vi "2DScatterFit2.vi"() -> ()   [LabVIEW 2014]
uses:
  <vilib>/Analysis/1siggen.llb/Ramp Pattern by Samples.vi
  <vilib>/gmath/NumericalOptimization/Nonlinear Curve Fit LM.vi
  <vilib>/Platform/NI_3dgraph.lvlib
  <vilib>/gmath/NI_Gmath.lvlib
  <vilib>/Analysis/NI_AALBase.lvlib
panel:
  in  "View":enum32{"2D", "3D"}(tab)=enum."3D"
  out "Z, Fit/Guess, Residual":dbl[][](graph)
  out "X,Y":dbl[][](graph)
  in  "3D Curve":refnum<k7>(container)
  in  "Fit!":bool
  out "Best Fit":dbl[](array[numeric]) format="%.2f"
  in  "Guess":dbl[](array[numeric])=[3.0, 10.0, -2.0, 10.0, 5.0] format="%.2f"
  out "Parameter Names":string[](array[string])=["Xposition", "Xwidth", "Yposition", "Ywidth", "Amplitude"]
  in  "stop":bool
  out "note":string
  # "Demo for NI-WEEK 2007\nChristian Altenbach\naltenbach@gmail.com"
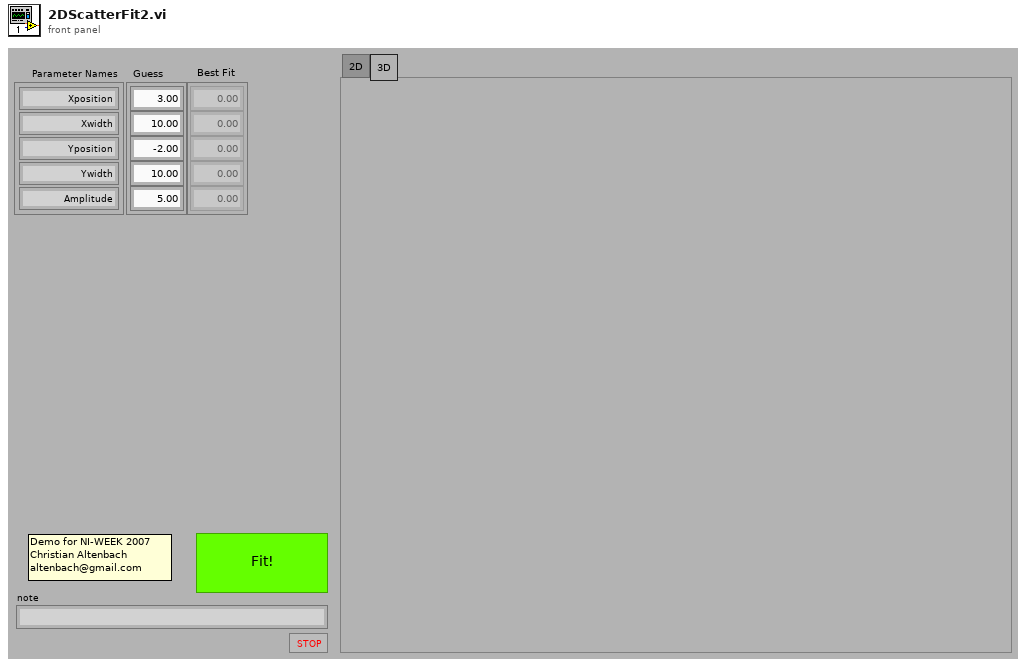
[diagram p1: front panel]
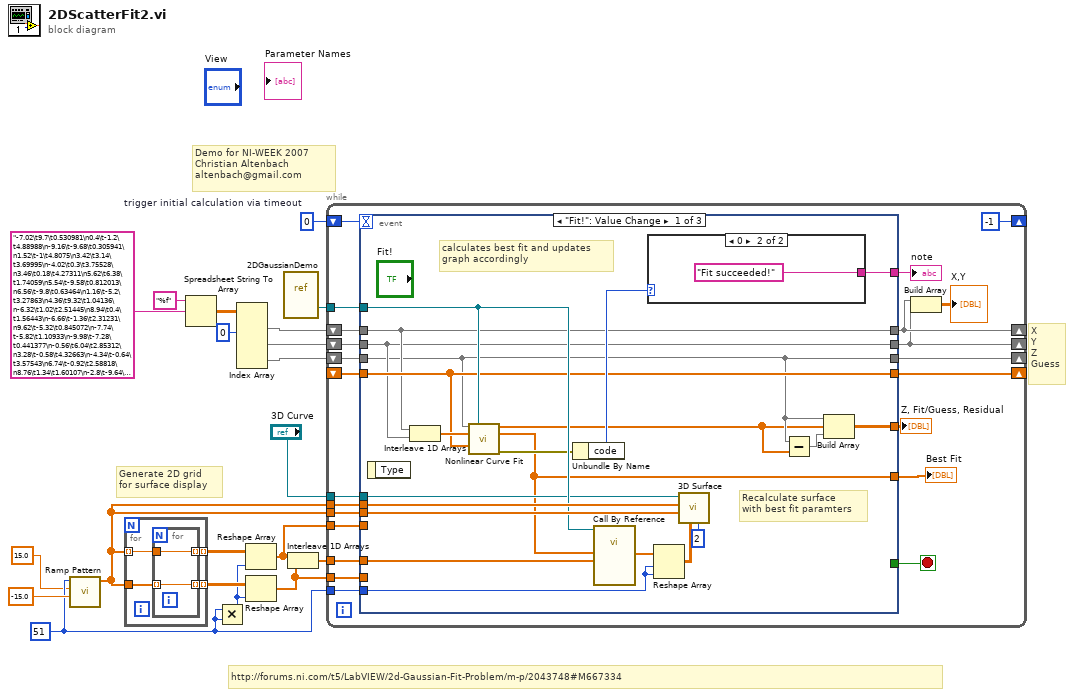
[diagram p0: block diagram]
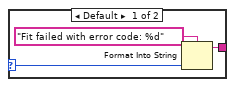
[diagram p2: hidden frame]
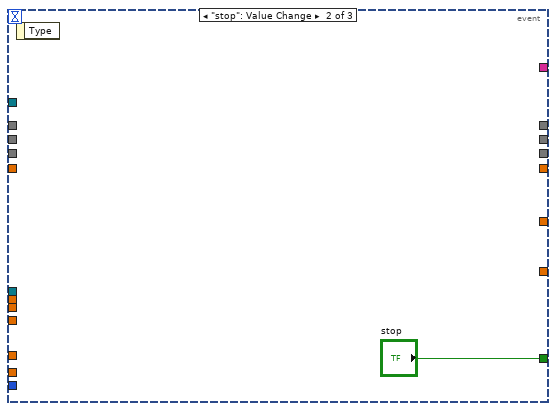
[diagram p3: hidden frame]
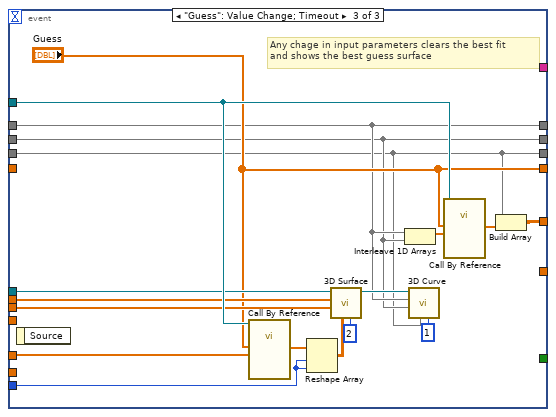
[diagram p4: hidden frame]
diagram:
  w14 = 0  # trigger initial calculation via timeout
  w16 = 51 ("samples")
  # "http://forums.ni.com/t5/LabVIEW/2d-Gaussian-Fit-Problem/m-p/2043748#M667334"
  # "Demo for NI-WEEK 2007\nChristian Altenbach\naltenbach@gmail.com"
  # "X\nY\nZ\nGuess"
  # "Generate 2D grid\nfor surface display"
  n1 = call-poly <vilib>:"Ramp Pattern.vi"("start"=-15.0, "end"=15.0, "samples"=w16) -> ("Ramp Pattern"=w8:dbl[])  [unwired: 7 in, 1 out]
  n2 = for {
    tunnel: w8 -> [w24] mode=indexing
    tunnel: w8 -> [w23]
    tunnel: [w22] -> w19 mode=indexing
    tunnel: [w21] -> w18 mode=indexing
    n3 = for {
      tunnel: w24 -> [w26]
      tunnel: w23 -> [w25] mode=indexing
      tunnel: [w26] -> w22 mode=indexing
      tunnel: [w25] -> w21 mode=indexing
    }
  }
  n4 = Spreadsheet String To Array(format string="%f", spreadsheet string="-7.02\t9.7\t0.530981\n0.4\t-1.2\t4.88988\n-9.16\t-9.68\t0.305941\n1.52\t-1\t4.8075\n3.42\t3.14\t3.69995\n-4.02\t0.3\t3.75528\n3.46\t0.18\t4.27311\n5.62\t6.38\t1.74059\n5.54\t-9.58\t0.812013\n6.56\t-9.8\t0.63464\n1.16\t-5.2\t3.27863\n4.36\t9.32\t1.04136\n-6.32\t1.02\t2.51445\n8.94\t0.4\t1.56443\n-6.66\t-1.36\t2.31231\n9.62\t-5.32\t0.845072\n-7.74\t-5.82\t1.10933\n-9.98\t-7.28\t0.441377\n-0.56\t6.04\t2.85312\n3.28\t-0.58\t4.32663\n-4.34\t-0.64\t3.57543\n6.74\t-0.92\t2.58818\n8.76\t1.34\t1.60107\n-2.8\t-9.64\t1.05793\n8.26\t-4.1\t1.44729\n5.88\t1.34\t2.99639\n0.68\t-1.06\t4.90224\n-6.74\t4.42\t1.7417\n4.4\t-6.82\t1.90029\n4.36\t-8.66\t1.24117\n4.62\t3.24\t3.18956\n3.4\t8.42\t1.47493\n8.46\t-9.42\t0.46356\n9.06\t-8.98\t0.447721\n-0.1\t8.6\t1.63387\n9.4\t-0.78\t1.36902\n-5.2\t-2.52\t2.85715\n-3.18\t-7.78\t1.66237\n-4.08\t-0.64\t3.70658\n3.18\t3.78\t3.53928\n7.86\t-6.78\t1.02478\n-5.44\t-3.16\t2.59411\n-7.94\t9.98\t0.391925\n6.6\t-1.12\t2.64428\n1.96\t7.26\t2.16044\n-0.86\t-3.3\t4.15442\n-2.28\t4.72\t3.23096\n-8.48\t-8.54\t0.507106\n1.48\t-1.14\t4.79288\n-2.56\t-6.28\t2.42944\n-7.78\t-1.96\t1.73096\n-0.12\t-1.6\t4.79692\n0.82\t-2.54\t4.51213\n6.32\t-0.22\t2.84146\n4.98\t-5.72\t2.16342\n3.52\t6.54\t2.22911\n4.34\t2.46\t3.53708\n-7.36\t-3.3\t1.72222\n-4.66\t7.86\t1.35106\n4.28\t-7.26\t1.75649\n6.4\t3.18\t2.40575\n-6.7\t-3.58\t1.94133\n-7.3\t3.08\t1.78659\n-5.94\t3.94\t2.1791\n-8.62\t-1\t1.45051\n-4.82\t0.8\t3.31652\n-3.58\t-5.66\t2.44563\n-5.26\t-3.06\t2.70188\n-6.32\t-0.66\t2.53662\n-4.84\t1.68\t3.19938\n-4.1\t6.08\t2.13012\n-1.78\t-1.34\t4.55738\n-2.32\t3.54\t3.73108\n0.1\t0.96\t4.92949\n-9.52\t-7.42\t0.493349\n6.34\t5.98\t1.65203\n-2.3\t0.98\t4.44901\n6.88\t-9.5\t0.649987\n9.6\t-1.72\t1.24779\n-9.04\t5.76\t0.793552\n-1.82\t-8.98\t1.37785\n2.34\t-7.8\t1.86285\n-7.5\t-2.46\t1.79252\n-6\t-5.16\t1.81762\n-6.56\t3.08\t2.10648\n3.4\t-2.04\t4.03612\n8.72\t-5.28\t1.08912\n7.32\t0.18\t2.32211\n7.92\t-3.52\t1.67987\n-3.08\t9.6\t1.04529\n-2.5\t4.24\t3.38577\n-7.24\t-1.42\t2.02639\n-4.1\t0.66\t3.69618\n-0.22\t-1.02\t4.90226\n8.32\t-9.62\t0.453237\n2.26\t-3.06\t4.08115\n1.84\t-5.08\t3.2556\n-1.16\t8.06\t1.81703\n0.48\t7.64\t2.07089\n-2.38\t-7.86\t1.75913\n0.08\t8.72\t1.58589\n-9.02\t8.62\t0.428851\n3.4\t0.26\t4.29596\n-9.24\t-8.94\t0.368135\n-5\t1.34\t3.16682\n3.14\t2.58\t3.9853\n-3.6\t2.74\t3.5415\n3.58\t-9.46\t1.08953\n0.98\t2.2\t4.61388\n-7.94\t1.82\t1.67746\n8.94\t-0.64\t1.55819\n7.92\t-2.48\t1.84647\n2.38\t-9.32\t1.25331\n4.74\t8.24\t1.31895\n0.32\t4.56\t3.65473\n5.64\t8.84\t0.9855\n-6.42\t-3.82\t2.0049\n-2.02\t-6.38\t2.48753\n-0.06\t2.68\t4.4803\n8.64\t-8.68\t0.542172\n-1.02\t-1.96\t4.59522\n-1.3\t-0.04\t4.81179\n7.2\t8.12\t0.881388\n-1.24\t1.92\t4.56605\n-7.1\t5.64\t1.33583\n3.76\t-0.96\t4.08675\n-8.6\t5.22\t0.982076\n7.96\t7.5\t0.859444\n-0.2\t-1.66\t4.77755\n0\t-7.24\t2.25744\n-8\t8.4\t0.598539\n-2\t4.88\t3.22355\n-6.04\t5.56\t1.69424\n4.36\t-6.98\t1.84718\n-1.64\t1.98\t4.45456\n0.84\t0.98\t4.90476\n-0.18\t6.64\t2.5628\n3.66\t1.7\t4.01154\n9.84\t0.36\t1.21478\n-1.68\t-7.36\t2.07473\n-8.28\t-9.08\t0.463232\n-5.22\t-9.38\t0.8276\n-4.22\t7.96\t1.40648\n2.34\t6.82\t2.32071\n-5.94\t-2.14\t2.56781\n4.66\t1.72\t3.55425\n-4.4\t-0.94\t3.51923\n-5.26\t0.28\t3.11132\n1.22\t-3.22\t4.21313\n-9.94\t6.84\t0.492513\n-1.34\t-1.88\t4.55075\n7.44\t-0.02\t2.26275\n-2.46\t7.1\t2.08189\n-2.02\t7.84\t1.823\n4.36\t-0.5\t3.84916\n2.26\t2.78\t4.18858\n-2.58\t-1.9\t4.1725\n5.22\t-3.4\t2.87572\n2.02\t7.56\t2.01372\n-8.9\t-4.5\t1.00198\n5.26\t9.28\t0.928388\n-1.34\t-4.98\t3.29733\n-8.96\t-3.36\t1.12821\n-4.14\t-4.92\t2.56328\n-4.66\t9.92\t0.776929\n-4.82\t-5.04\t2.278\n0.84\t-8.86\t1.5156\n8.42\t8.38\t0.621874\n-7.86\t-0.58\t1.78954\n1.68\t-1.68\t4.64565\n-9.28\t5.52\t0.77081\n-9.44\t-7.76\t0.467417\n1.78932e-307\t7.18\t2.29428\n-5\t-3.06\t2.82177\n-9.88\t4.02\t0.796954\n-5.74\t-6.44\t1.52521\n-6.74\t-7.48\t1.00177\n2.04\t-7.3\t2.12571\n-1.6\t1.08\t4.65393\n1.38\t9.28\t1.33725\n-3.64\t4.9\t2.74756\n-0.34\t-2.5\t4.52021\n4.9\t1.08\t3.53143\n3.74\t6.14\t2.35232\n3.64\t3.62\t3.44611\n-5.26\t-6.82\t1.53957\n9.04\t-1.62\t1.46654\n3.26\t1.1\t4.27932\n9.46\t-1.92\t1.28447\n4.18\t-8.36\t1.37098\n0.12\t-2.64\t4.49572\n-8.22\t1.04\t1.61376\n-1.82\t7.7\t1.90962\n-5.2\t-5.24\t2.07535\n-2.4\t-7.62\t1.8578\n-8.78\t2.8\t1.25228\n4.24\t1.76\t3.74421\n3.54\t-5.6\t2.63663\n-9.2\t7.88\t0.489488\n-6.56\t-6.74\t1.22082\n-8.04\t-0.3\t1.71602\n-2.8\t-7.58\t1.80952\n-0.84\t-1.86\t4.65302\n0.32\t9.36\t1.33229\n-4.24\t-9.12\t1.0357\n-7.3\t0.76\t2.04315\n-8.02\t7.6\t0.7225\n3.72\t-2.14\t3.88248\n-0.02\t-5.3\t3.26176\n-3.06\t1.22\t4.118\n8.7\t-9.42\t0.43588\n5.5\t-4.28\t2.48422\n-1\t0.5\t4.85807\n6.78\t5.7\t1.59355\n-1.38\t-8.48\t1.61302\n-2.46\t9.8\t1.04498\n-2.8\t7.68\t1.77408\n9.06\t-3.94\t1.19958\n1.18\t4.78\t3.49872\n1.76\t-3.06\t4.19197\n8.98\t5.58\t0.970049\n0.64\t4.22\t3.81545\n5.74\t-5.32\t2.05272\n10\t4.06\t0.905243\n-1.36\t-6.42\t2.56925\n8.48\t-8\t0.670589\n-8.36\t-4.34\t1.18762\n4.12\t8.04\t1.50018\n0.62\t1.12\t4.89826\n9.38\t-8.68\t0.44404\n8.32\t-7.94\t0.708242\n-4\t-4.34\t2.83319\n-0.7\t7.52\t2.09889\n-9.78\t4.08\t0.816216\n-4.92\t-1.72\t3.15008\n7.58\t3.94\t1.73579\n9.04\t2.14\t1.42498\n7.96\t2.06\t1.88441\n1.36\t-1.34\t4.77709\n-9.38\t-0.36\t1.18229\n-5.84\t4.38\t2.10161\n9.36\t7.22\t0.63646\n6.5\t7.62\t1.14429\n7.12\t-0.32\t2.42109\n9.16\t3.62\t1.21274\n-8.66\t-8.64\t0.470379\n-0.14\t9.5\t1.27683\n8.88\t-9.08\t0.457232\n-1.74\t-0.8\t4.64992\n0.82\t-3.56\t4.10614\n0.86\t-1.34\t4.83907\n-2.26\t-9.74\t1.07659\n-4.04\t0.56\t3.73287\n-5.4\t-5.74\t1.84518\n-1.16\t-0.48\t4.82604\n5.68\t4.6\t2.31489\n6.6\t7.04\t1.27612\n-0.38\t6.78\t2.48257\n-6.82\t6.44\t1.229\n-5.52\t-9.28\t0.807905\n4.52\t7.98\t1.44792\n-7.3\t5.78\t1.24511\n-6.72\t3.78\t1.89343\n-3.94\t-4.42\t2.82543\n-5.88\t2.8\t2.47513\n0.76\t-6.82\t2.46242\n-1.5\t5.92\t2.80718\n-7.7\t-4\t1.46848\n9.8\t0.86\t1.21804\n0.66\t0.88\t4.93146\n-1.8\t-2.76\t4.16679\n-4.94\t-1.08\t3.22664\n-4.14\t1.54\t3.5708\n-0.74\t-9.32\t1.32085\n-8.24\t-7.9\t0.633937\n6.24\t1.16\t2.82878\n6.78\t-5.8\t1.56221\n-6.58\t-5.46\t1.53981\n8.6\t-5.08\t1.15931\n-2.34\t9.62\t1.11263\n6.86\t-1.76\t2.44135\n-9.94\t-5.7\t0.609686\n8.04\t0.04\t1.97037\n-8.76\t1.12\t1.39063\n-9.54\t3.04\t0.982464\n6.08\t1.84\t2.82423\n-0.56\t-8.18\t1.79549\n-1.14\t2.62\t4.37226\n2.04\t7.94\t1.84031\n8.28\t-1\t1.83024\n2.24\t4.7\t3.3766\n2.36\t-9.08\t1.34164\n-4.1\t2.34\t3.42625\n-6.46\t-2.3\t2.28934\n5.78\t2.98\t2.7396\n-6.38\t-7.04\t1.19061\n-3.56\t5.6\t2.48263\n8.8\t-0.2\t1.62641\n9.44\t1.06\t1.34367\n-5.46\t5.62\t1.86836\n-1.96\t7.1\t2.16336\n-9.16\t-2.82\t1.12022\n2.56\t3.32\t3.90749\n-3\t-4.32\t3.19202\n5.08\t6.22\t1.95291\n6.66\t-8.32\t0.933789\n4.58\t4.14\t2.90085\n2.86\t0.12\t4.50896\n-8.1\t-7.7\t0.689307\n-6.98\t-4.78\t1.56816\n4.84\t7.9\t1.41309\n3.98\t5.76\t2.4525\n2.92\t4.8\t3.17122\n-3.14\t9.7\t1.0089\n2.7\t8.94\t1.36649\n2.24\t9.48\t1.21308\n-7.52\t-7\t0.931012\n-4.98\t6.9\t1.59128\n7.56\t-8.36\t0.764436\n9.56\t-1.86\t1.25265\n5\t-3.66\t2.89028\n-5.6\t8.78\t0.916387\n-1.22\t-9.58\t1.20359\n7.74\t8.68\t0.678151\n-5.22\t4.18\t2.41026\n-8.14\t7.16\t0.772657\n5.76\t9.68\t0.763586\n8.7\t7.9\t0.651396\n6.28\t-4.12\t2.2145\n-5.7\t3.94\t2.27983\n7.86\t3.7\t1.6732\n-5.7\t-7.32\t1.27926\n-6.2\t0.82\t2.59037\n-1.42\t-9.04\t1.38761\n-5.6\t-3.12\t2.53047\n-3.56\t9.98\t0.885656\n1.78\t-1.62\t4.63875\n-8.46\t-9.82\t0.357291\n4.88\t3.64\t2.95183\n-3.04\t-3.42\t3.5328\n4.56\t-2.08\t3.52554\n-9.9\t-6.6\t0.522166\n8.56\t8.34\t0.606263\n7.8\t-0.6\t2.07371\n6.5\t-1.16\t2.69229\n1.14\t2.56\t4.47883\n4.86\t5.32\t2.35856\n-9.28\t-4.7\t0.873001\n2\t-9.52\t1.21076\n1.5\t9.48\t1.25812\n3.16\t-1.02\t4.3274\n-2.28\t-8.84\t1.38434\n-4.58\t-7.74\t1.40204\n-1.94\t-4\t3.63595\n2.82\t3.72\t3.67302\n-9.42\t3.88\t0.933114\n1.18\t-6.48\t2.61318\n7.74\t-5.94\t1.23873\n-6.78\t3.88\t1.84746\n1.26\t0.28\t4.92015\n3.6\t-6.34\t2.29253\n-2.66\t5.56\t2.7461\n-6.26\t-6.2\t1.44374\n-8.46\t-2.72\t1.3749\n-2.94\t2.06\t3.99896\n3.8\t2.3\t3.81171\n-6.24\t-2.04\t2.43612\n-6.64\t1.76\t2.28036\n5.98\t-1.96\t2.85279\n-6.06\t6.2\t1.50633\n-7.36\t-9.36\t0.53925\n8.62\t-9.48\t0.437436\n4.7\t-9\t1.08385\n4.72\t9.12\t1.05003\n-0.22\t-3.74\t4.0284\n9.12\t-9.46\t0.385258\n-2.44\t0.38\t4.45242\n2.92\t-7.1\t2.09124\n-5.48\t9.22\t0.830769\n-3.28\t-1.36\t3.99856\n-1\t-4.54\t3.56697\n5.48\t9.54\t0.832893\n6.28\t-6.2\t1.60008\n3.42\t1.7\t4.10981\n-6.62\t-4.32\t1.80755\n-0.78\t0.76\t4.87278\n-5.64\t4.48\t2.15221\n-9.04\t-3.42\t1.09587\n-4.94\t-9.62\t0.809049\n1.06\t-1.5\t4.78549\n8.22\t5.58\t1.17943\n-8.7\t-9.84\t0.332602\n8.44\t-1.04\t1.75636\n-2.14\t4.68\t3.28446\n7.18\t-8.56\t0.789354\n6.3\t-0.62\t2.83738\n7.84\t-9.24\t0.567122\n6.52\t-8.92\t0.820607\n0.62\t6.54\t2.6179\n7.82\t-9\t0.608791\n-2.34\t5.22\t2.98308\n-6.16\t-0.32\t2.63306\n7.96\t5.18\t1.34015\n-2.28\t2.02\t4.25171\n-7.7\t-8.38\t0.64629\n-3.2\t2.3\t3.83204\n-1.5\t-8.3\t1.67774\n7.92\t-0.8\t2.00762\n-3.86\t9.44\t1.00007\n2.2\t0.8\t4.67731\n-8.32\t0.6\t1.58881\n0.24\t-0.52\t4.97894\n3.54\t7.98\t1.62222\n6.94\t7.08\t1.18185\n-3.14\t-3.88\t3.32287\n6.6\t9.74\t0.643683\n-1.16\t6.62\t2.50048\n-2.12\t3\t3.99639\n-6.6\t-7.28\t1.07948\n8.86\t6.82\t0.79409\n-3.56\t-5.26\t2.61902\n-8.12\t0.44\t1.67859\n-9.32\t-5.24\t0.795395\n-1.14\t-2.42\t4.43458\n0.74\t-8.26\t1.77327\n-4.12\t1.3\t3.61743\n8.1\t-3.42\t1.62616\n-1.46\t-1.04\t4.69428\n6.1\t7.02\t1.40762\n6.74\t-2.6\t2.36597\n-5.02\t2.62\t2.92445\n-0.26\t-2.2\t4.62447\n-3.14\t-0.12\t4.17461\n-8.76\t-9.34\t0.378173\n-9.28\t7.2\t0.558207\n4.34\t-9.04\t1.1239\n7.46\t-0.26\t2.25034\n6.4\t-7.04\t1.32213\n4.76\t-5.34\t2.37866\n4.22\t5.36\t2.54954\n2.22\t5.98\t2.75021\n-1.02\t6.18\t2.73858\n-3.64\t-0.52\t3.92925\n1.24\t-2.18\t4.5848\n-4.48\t7.96\t1.35518\n5.9\t2.14\t2.86344\n-5.04\t5.96\t1.89136\n7.28\t-4.76\t1.66202\n-8.24\t5.04\t1.11237\n-5.98\t2.74\t2.44034\n-0.04\t8.52\t1.6691\n4.22\t-5.5\t2.48578\n5.34\t6.62\t1.73694\n0.24\t-0.12\t4.99868\n0.68\t-8.56\t1.64424\n3.94\t2.5\t3.699\n0.56\t-7.96\t1.91274\n-8.6\t-4.6\t1.07449\n-3.5\t9.26\t1.09955\n8.3\t-3.96\t1.45775\n-8.16\t-9.28\t0.452217\n4.44\t1.22\t3.74084\n-3.16\t6.2\t2.33341\n9.2\t2.08\t1.36924\n3.58\t2.04\t3.9681\n6.18\t-0.82\t2.88809\n1.04\t-3.32\t4.19146\n8.48\t-2.56\t1.60012\n-9.92\t-4.66\t0.722246\n-6.54\t1.16\t2.39145\n-1.52\t5.14\t3.19419\n-1.98\t9.02\t1.3536\n-4.22\t1.78941e-307\t3.65941\n-6.76\t9.06\t0.674288\n8.54\t5.88\t1.03355\n-0.28\t-6.34\t2.70637\n-4.96\t-4.6\t2.37544\n2.36\t-5.32\t3.04433\n0.58\t3.28\t4.24635\n5.46\t-1.72\t3.15554\n-7.78\t-9.08\t0.526637\n7.7\t-0.02\t2.13399\n-6.02\t-8.26\t0.964655\n-2.92\t-0.26\t4.26589\n1.72\t5.98\t2.82314\n6.1\t-3.2\t2.53432\n-1.86\t-4.34\t3.5019\n6.5\t4.9\t1.91372\n7.9\t-0.16\t2.03621\n4.46\t7.04\t1.80614\n-7.58\t9.38\t0.510769\n-4.48\t-9.38\t0.930474\n5.12\t1.98\t3.28079\n-0.34\t2.54\t4.51135\n6.2\t-2.74\t2.59397\n-3.9\t3.86\t3.0518\n-2.24\t-8.3\t1.59745\n-1.44\t5.18\t3.18814\n-1.18\t-6.32\t2.64188\n-9.94\t1.4\t0.968784\n0.22\t-1.56\t4.81753\n-1.94\t6.86\t2.27878\n-0.3\t3.08\t4.31272\n9.34\t-9.86\t0.32251\n-3.14\t1.56\t4.02614\n5.04\t9.42\t0.922446\n8.22\t-0.26\t1.88416\n-4.28\t7.02\t1.72527\n2.06\t-9.62\t1.17239\n-3.68\t4.76\t2.79062\n-6.32\t8.12\t0.944109\n1.14\t-1.2\t4.83491\n0.18\t4.36\t3.75407\n-1.18\t-5.28\t3.17118\n-4.48\t2.52\t3.20492\n7.46\t2.46\t2.0569\n5.62\t-7.2\t1.46659\n9.44\t-8.78\t0.425202\n3.14\t7.38\t1.93647\n6.56\t4.8\t1.91957\n2.72\t-4.88\t3.17734\n-5.04\t-3.86\t2.57784\n-4.16\t-3\t3.21834\n0.28\t2.74\t4.46614\n5.88\t0.7\t3.0557\n-7.64\t1.34\t1.84939\n3.06\t-4.18\t3.40285\n0.54\t3.14\t4.30583\n-0.54\t8.9\t1.49713\n8.48\t8.68\t0.566952\n4.12\t-1.8\t3.78772\n9.22\t2.88\t1.28264\n-2.14\t9.08\t1.31629\n0.16\t-10\t1.09991\n8.46\t8.54\t0.590964\n-1.86\t8.82\t1.44023\n5.46\t0.6\t3.28362\n-5.7\t7.3\t1.28898\n-4.64\t1.14\t3.37654\n9.24\t-2.16\t1.34603\n-3.44\t-7.14\t1.86628\n7.8\t-7.72\t0.845532\n-5.72\t0.44\t2.86169\n-5.7\t-3.18\t2.47039\n-4.38\t5.28\t2.34984\n7.5\t7\t1.06605\n4.58\t0.78\t3.7218\n-4.68\t2.66\t3.07639\n-3.02\t7.18\t1.94227\n-9.76\t3.18\t0.906395\n-4.4\t6.58\t1.85642\n4.1\t2.2\t3.70917\n5.04\t-2.08\t3.29677\n3.02\t2.78\t3.96239\n6.78\t-7.88\t1.01558\n2.54\t-7.68\t1.89051\n-5.88\t6.94\t1.34656\n2.58\t-2.36\t4.23207\n7.42\t1.9\t2.15296\n2.48\t-0.08\t4.63786\n8.68\t-6.46\t0.892338\n-4.14\t9.68\t0.899211\n-3.1\t-9.8\t0.979579\n5.84\t1.84\t2.9458\n3\t7.18\t2.04814\n-0.26\t-9.32\t1.33612\n4.68\t1.48\t3.58583\n4.46\t4.98\t2.62505\n1.52\t7.16\t2.2524\n1.08\t2.66\t4.4506\n-9.98\t-10\t0.216745\n0.22\t6.2\t2.79987\n-1.42\t2.86\t4.22912\n-3.26\t-2.64\t3.70781\n2.4\t0.26\t4.65877\n5.02\t-7.66\t1.45208\n-1.42\t-6.32\t2.6112\n-6.38\t-3.28\t2.14239\n1.12\t6.56\t2.58372\n0.7\t0.38\t4.97563\n-4.12\t9.04\t1.08056\n8.62\t-7.4\t0.744114\n-4.42\t-6.76\t1.77993\n-0.84\t-2.9\t4.31652\n-5.14\t8.24\t1.14081\n8.56\t6.92\t0.841018\n5.2\t-5.24\t2.26734\n2.28\t-0.58\t4.67467\n9.92\t0.66\t1.18089\n-9.72\t-8.56\t0.352277\n-0.74\t-4.52\t3.60983\n1.92\t-5.82\t2.86999\n5.38\t5.72\t2.04123\n0.78\t8.18\t1.81422\n-2.8\t9.76\t1.02563\n-0.06\t-1.7\t4.77618\n-4.38\t-7.24\t1.61713\n-3.16\t8.9\t1.26053\n8.42\t1.92\t1.69815\n8.26\t-1.38\t1.81418\n5.1\t1.18\t3.41821\n5.38\t-4.48\t2.46594\n-7.82\t6.42\t0.975754\n8.72\t-8\t0.630453\n8.12\t0.34\t1.92953\n3.22\t-0.08\t4.37278\n-2\t7.6\t1.93066\n-6.82\t5.4\t1.48015\n9.04\t9.64\t0.375333\n-2.72\t3.98\t3.42886\n5.18\t-0.2\t3.4461\n3.58\t-4.42\t3.14072\n2.28\t-1.62\t4.51472\n4.46\t-0.46\t3.80255\n3.08\t7.48\t1.90346\n-8.3\t9.52\t0.408797\n-7.82\t6.02\t1.0519\n-8.46\t8.54\t0.511735\n-8.92\t4.92\t0.940374\n-0.48\t4.02\t3.88518\n-6.86\t1.9\t2.15733\n-4.5\t2.76\t3.13502\n-1.38\t-3.46\t3.99631\n-1.16\t5.98\t2.8243\n9.58\t5.4\t0.845806\n3.18\t4.16\t3.38174\n5\t-3.26\t3.01406\n-8.46\t-7.76\t0.618011\n-4.24\t5.88\t2.16642\n-8.6\t4.58\t1.07961\n-0.38\t9.88\t1.13786\n9.58\t9.78\t0.309832\n-3.84\t2.72\t3.4438\n7.16\t5.9\t1.42241\n1.88\t-9.72\t1.14936\n-5.3\t-4.64\t2.23181\n5.12\t5.32\t2.27092\n7.2\t-0.02\t2.38407\n1.1\t2.4\t4.53747\n-1.14\t-4.1\t3.75643\n7\t-6.98\t1.18875\n-1.56\t8.74\t1.49844\n-3.3\t0.56\t4.08519\n3.94\t8.32\t1.42942\n-3.86\t-4.78\t2.7151\n-2.22\t3.98\t3.57739\n-1.96\t9.18\t1.29714\n1.78\t-0.6\t4.80136\n-3\t-8.7\t1.34654\n-7.92\t7.66\t0.73096\n4.52\t2.56\t3.43024\n-5.74\t6.1\t1.63116\n3.94\t-9.4\t1.06622\n-1.78\t-8.44\t1.59268\n5.48\t5.14\t2.20943\n-6.74\t-4.76\t1.65813\n1.26\t-7.46\t2.12015\n3.08\t-2.36\t4.06833\n0.3\t-8.76\t1.56421\n0.68\t3.74\t4.04\n3.42\t6.48\t2.27794\n3.52\t-2.24\t3.93729\n-1.64\t5.32\t3.08339\n8.38\t-1.58\t1.74511\n-5.28\t-8.24\t1.11011\n6.42\t-6.26\t1.54105\n-0.96\t1.68\t4.68121\n-1.8\t-3.8\t3.75759\n9.64\t-2.2\t1.19874\n8.66\t-2.46\t1.53967\n-8.3\t4.74\t1.14448\n2.06\t3.96\t3.75849\n-7.58\t3.96\t1.52211\n-2.92\t-9.06\t1.23219\n-4.26\t8.84\t1.11872\n1.82\t-1.48\t4.66064\n-2.46\t-0.4\t4.44314\n8.64\t5.92\t1.00019\n0.54\t-1.64\t4.79388\n9.36\t6.82\t0.6928\n9.36\t4.1\t1.08486\n-9.9\t4.26\t0.768565\n5.44\t7.7\t1.35356\n6.52\t5.7\t1.67727\n2.2\t6.86\t2.32155\n-1.56\t-2.12\t4.43266\n-0.18\t1.2\t4.87794\n5.22\t2.02\t3.22377\n0.46\t7.24\t2.26596\n0.48\t8.66\t1.61097\n3.1\t-6.74\t2.221\n7.32\t-7.32\t1.03176\n-1.46\t-5.42\t3.05758\n-6.9\t8.46\t0.766415\n4.6\t8.28\t1.3309\n4.68\t4.58\t2.70105\n0.82\t8.32\t1.75087\n3.2\t-0.86\t4.3317\n3.72\t0.58\t4.14213\n-0.8\t-5.46\t3.1258\n1.64\t-2.22\t4.50725\n7.62\t-7.42\t0.943918\n9.84\t-5.46\t0.774579\n2.74\t9.5\t1.16559\n5.38\t2.38\t3.07052\n-6.76\t-9.3\t0.628339\n2.3\t4.6\t3.4117\n-2.82\t6.24\t2.39675\n6.44\t-8.56\t0.916528\n-3.04\t5.36\t2.73592\n-9.5\t-4.96\t0.786996\n-5.62\t-8.3\t1.02974\n9.18\t4.4\t1.09744\n5.66\t-1.62\t3.06971\n-6.16\t0.32\t2.63343\n-3.76\t2.78\t3.46139\n7.96\t-9.44\t0.521018\n-3.84\t1.7\t3.6859\n1.68\t4.78\t3.43688\n-5.36\t6.32\t1.67601\n7.18\t9.4\t0.63081\n-4.62\t-2.86\t3.04958\n-6.64\t2.78\t2.12664\n-8.58\t-0.84\t1.4731\n1.18\t-9.84\t1.13976\n0.2\t-3.38\t4.20343\n-1.68\t-1.28\t4.59667\n-1.52\t8.24\t1.70731\n-5.62\t-7.66\t1.20187\n-2.54\t2\t4.16604\n-4.14\t6.98\t1.77401\n-2.32\t-9.64\t1.10336\n1.14\t5.28\t3.24641\n4.08\t5.16\t2.6763\n-4.58\t-8.14\t1.27355\n0.92\t-7.52\t2.10948\n5.84\t8.3\t1.09576\n6.92\t7.98\t0.967029\n-3.66\t7.86\t1.54946\n-9.96\t-8.56\t0.326825\n2.82\t-9.22\t1.24887\n2.8\t2.28\t4.19081\n8.02\t-0.74\t1.96323\n-3.06\t-5.9\t2.48447\n-3.52\t-7.82\t1.58522\n-1.34\t1.78941e-307\t4.80247\n9.78\t0.46\t1.23494\n3.52\t-2.64\t3.82247\n1.22\t1.82\t4.69252\n-8.64\t3\t1.27932\n-8.98\t-4.16\t1.02408\n1.58\t8.1\t1.80936\n1.36\t-0.94\t4.84383\n7.8\t3.14\t1.79774\n-8.84\t-0.2\t1.38459\n-6.96\t3.12\t1.92388\n-8.7\t-6.72\t0.726872\n4.8\t2.32\t3.36141\n-0.46\t-3.34\t4.18584\n9.82\t9.4\t0.322552\n-4.54\t3.9\t2.77922\n9.26\t2.38\t1.31982\n-4.46\t0.84\t3.49942\n-6.32\t3.72\t2.07332\n8.16\t0.24\t1.9125\n-1.96\t-4.8\t3.26379\n8.54\t-3.3\t1.47564\n-3.4\t-6.98\t1.94003\n-6.24\t1.7\t2.48541\n-1.96\t2.7\t4.14799\n-2.12\t-1.4\t4.44099\n0.42\t-5.84\t2.98091\n6.72\t-2.34\t2.42214\n6.16\t-3.3\t2.4824\n-7.04\t-9.06\t0.631239\n-3\t-6\t2.45511\n-8.7\t7.5\t0.616544\n9.22\t-0.88\t1.43591\n-6.82\t8.12\t0.849383\n8.26\t9.48\t0.480976\n1.98\t0.54\t4.76009\n4.1\t1.82\t3.79551\n7.9\t-5.58\t1.27071\n6.02\t7.36\t1.32624\n3.06\t-3.78\t3.57097\n-2.32\t6.66\t2.30768\n-3.54\t4.32\t3.01432\n-7.84\t4.6\t1.31426\n8.98\t3.9\t1.23369\n6.9\t5.5\t1.60874\n8.3\t2.12\t1.72865\n-1.4\t8.04\t1.80495\n4.04\t2.94\t3.52717\n-1.48\t0.24\t4.76369\n2.72\t2.24\t4.22812\n7.2\t-5.44\t1.52232\n2.66\t2.72\t4.09736\n9.52\t2.78\t1.18907\n9.16\t9.04\t0.430273\n9.8\t-8.96\t0.365158\n9.24\t2.62\t1.30337\n6.72\t-5.06\t1.78561\n6.94\t-3.14\t2.16767\n8.32\t-5.64\t1.13625\n-1.92\t-8\t1.76065\n7\t8.66\t0.801742\n5.46\t-9.86\t0.757539\n-5.44\t-8.6\t0.984989\n-6.38\t-9.74\t0.599852\n-2.78\t5.76\t2.6245\n4.12\t3.24\t3.3978\n-9.52\t-0.96\t1.11996\n-9.78\t6.78\t0.524244\n-5.7\t-1.88\t2.72946\n-7.76\t0.5\t1.83763\n7.96\t4.14\t1.5513\n-7.76\t0.9\t1.82229\n5.1\t7.64\t1.44644\n9.28\t-3.7\t1.16101\n8.8\t3.56\t1.34472\n-5.92\t2\t2.60269\n6.48\t6.18\t1.55077\n4.52\t-4.94\t2.6147\n4.92\t4.2\t2.74685\n0.1\t9.5\t1.27963\n5.32\t-4.4\t2.51616\n-2.62\t-8.9\t1.32379\n-1.82\t2.9\t4.11689\n4.68\t-7.32\t1.64563\n-1.54\t7.84\t1.87941\n-2.76\t8.86\t1.3261\n0.48\t6.6\t2.58999\n-7.84\t-8.98\t0.533175\n-7.16\t4.7\t1.52588\n3.48\t2.64\t3.8421\n-6.34\t-7.92\t0.983582\n-3.04\t-6.14\t2.38304\n5.34\t-1.92\t3.18072\n5.44\t-3.16\t2.84569\n9.64\t6.34\t0.703698\n3.46\t0.56\t4.25533\n2.76\t9.88\t1.04127\n2.52\t5.88\t2.74608\n-9.78\t6.14\t0.593971\n6\t0.5\t3.00296\n2.02\t-8.1\t1.76607\n4.12\t-5.94\t2.33129\n7.4\t-1.6\t2.19541\n8.98\t-6.96\t0.744724\n1.78932e-307\t6.14\t2.82817\n9.56\t-4.18\t1.01299\n2.92\t0.02\t4.48801\n6.74\t7.62\t1.09171\n3.56\t4.36\t3.1783\n8.26\t-4.5\t1.37383\n8.74\t-2.16\t1.53997\n3.68\t3.54\t3.46152\n9.6\t8.5\t0.43867\n-0.46\t7.52\t2.11224\n6.7\t8.76\t0.82998\n-5.82\t-9.84\t0.650245\n4.94\t-9.62\t0.879994\n-7.18\t-3.84\t1.69412\n8.68\t-0.4\t1.67514\n2.62\t6.98\t2.2022\n-3.5\t-8.08\t1.49258\n7.52\t-4.12\t1.71819\n-3.48\t7.32\t1.79159\n3.36\t3.24\t3.68573\n1.16\t5.02\t3.37853\n-7.1\t-8.96\t0.639915\n2.2\t-1.28\t4.60517\n0.78\t-1.64\t4.78023\n5.8\t-8.54\t1.03413\n8.46\t-4\t1.39377\n7.5\t-9.3\t0.602694\n9.28\t1.74\t1.3657\n7.24\t3.24\t2.01825\n3.46\t-4.86\t2.98814\n4.32\t-9.84\t0.896541\n-6.86\t-7.28\t1.02042\n-7.62\t2.14\t1.78215\n-2.66\t2.84\t3.87684\n-5.48\t-6.04\t1.72453\n6.88\t0.72\t2.52946\n-1.86\t0.04\t4.65988\n-0.54\t3.46\t4.13266\n-10\t9\t0.288221\n-5.26\t5.08\t2.1109\n-8.66\t-1.14\t1.4281\n9.24\t-8.62\t0.469042\n-7.34\t-7.94\t0.785718\n-8.82\t-4.84\t0.976748\n8.92\t-9.56\t0.395109\n-4.06\t-9.02\t1.09104\n-5.68\t-9.88\t0.659494\n0.58\t-9.64\t1.22259\n-2.34\t-3.32\t3.80542\n-0.94\t-3.34\t4.12574\n-3.1\t0.02\t4.19317\n-2.76\t0.08\t4.33641\n-5.5\t9.46\t0.773606\n7.92\t-7.26\t0.912445\n-7.76\t8.64\t0.597754\n5.62\t3.66\t2.62874\n6.32\t-9.42\t0.741936\n1.86\t-6.36\t2.60582\n2.24\t-7.2\t2.14798\n0.02\t-9.56\t1.25187\n9.96\t-7.98\t0.447669\n-9.7\t3.72\t0.872886\n-1.26\t-0.54\t4.79944\n4.86\t-0.1\t3.6133\n-7.72\t-4.38\t1.39246\n-7.38\t-2.66\t1.81611\n3.66\t5.46\t2.67239\n-5.5\t1.32\t2.9101\n-9.78\t-6.78\t0.522713\n-1.8\t-1.1\t4.59228\n8.86\t-2.36\t1.47175\n-6.68\t-5.9\t1.39748\n-9.38\t6.74\t0.596992\n6.4\t2.78\t2.49383\n-3.84\t-7.1\t1.79353\n-4.3\t7.66\t1.49281\n-9.66\t8.02\t0.41233\n6.56\t-6.7\t1.37614\n-2.48\t-1.84\t4.22318\n6.04\t1.3\t2.91801\n-3.7\t-1.06\t3.85018\n-1.9\t4.92\t3.22664\n-5.24\t-9.78\t0.734488\n-1.36\t4.44\t3.56458\n5.36\t-8.64\t1.08293\n-9.64\t1.96\t1.0338\n-0.2\t-3.98\t3.91809\n-2.08\t-3.56\t3.78624\n4.34\t7.24\t1.75654\n2.78\t-1.22\t4.43613\n-5.54\t-7.62\t1.23071\n-1.72\t6.7\t2.38862\n-9.86\t-1.66\t0.980929\n4.68\t-0.2\t3.70298\n-9.34\t6.26\t0.663843\n4.06\t-5.44\t2.55902\n9.72\t6.64\t0.648266\n-4.58\t-0.64\t3.45208\n-9.74\t-5.6\t0.660201\n9.66\t9.44\t0.334174\n-0.18\t3.92\t3.95414\n4.44\t1.86\t3.63151\n5.16\t3.8\t2.78271\n-0.6\t-9.36\t1.31135\n7.42\t-7.92\t0.878953\n-8.96\t1.66\t1.28497\n-2.84\t-8.76\t1.34646\n7.74\t7.64\t0.876334\n9.36\t3.08\t1.21162\n4.66\t3.16\t3.19701\n-1.8\t3.7\t3.80659\n-1.04\t-0.28\t4.86208\n-7.56\t-1.32\t1.88617\n4.64\t0.68\t3.7001\n-9.88\t-2.04\t0.954219\n7.54\t-3.72\t1.79371\n-6.32\t-9.2\t0.708894\n0.36\t-1.36\t4.86015\n4.88\t0.94\t3.55658\n-2.24\t-3.26\t3.85871\n-0.14\t1.36\t4.8506\n-8.82\t-8.6\t0.454598\n4.24\t9.52\t0.998524\n4.04\t-9.6\t0.995162\n7.9\t2.16\t1.89922\n6.54\t3.38\t2.29626\n0.12\t-9.5\t1.27452\n-9.26\t-3.28\t1.04258\n4.62\t-4.9\t2.59566\n5.74\t8.9\t0.953695\n-5.62\t0.88\t2.88953\n-7.74\t5.04\t1.26385\n6.92\t-7.92\t0.977719\n-1.84\t-7.7\t1.90082\n-1.04\t7.46\t2.10213\n-7.04\t-5.32\t1.42451\n1.7\t-5.04\t3.29686\n3.22\t8.06\t1.64066\n-4.34\t7.12\t1.67452\n7.24\t-4.9\t1.64245\n5.8\t-4.38\t2.33272\n-9.76\t0.48\t1.05184\n-3.62\t6.74\t1.99316\n-0.58\t5.64\t3.06007\n6.12\t-4.08\t2.29166\n-1.32\t3.96\t3.7958\n3.02\t3.18\t3.82244\n3.92\t-4.36\t3.05242\n-0.48\t7.76\t1.9975\n-2.16\t2.86\t4.03409\n7.44\t3.34\t1.91297\n5.08\t4.54\t2.56575\n") -> (array=w5:dbl[][])  [unwired: 2 in]
  n5 = Multiply(x=w16, y=w16) -> (x*y=w17:i32)
  n6 = Index Array(array=w5, index (col) #1=0 ("disabled index (col)")) -> (element #1=w3:dbl[], element #2=w2:dbl[], element #3=w1:dbl[])  [unwired: 5 in]
  n7 = Reshape Array(w19, w17) -> (w11:dbl[])
  n8 = Reshape Array(w18, w17) -> (w10:dbl[])
  n9 = vi-ref "2DGaussianDemo.vi"() -> (w13:refnum<vi>)
  n10 = Interleave 1D Arrays(w11, w10) -> (w15:dbl[])
  n11 = while {
    tunnel: w8 -> [w49]
    tunnel: w8 -> [w48]
    tunnel: w16 -> [w47]
    tunnel: w15 -> [w44]
    shift-right: [-1] -> _
    shift-left: w14 -> [w41]
    tunnel: w13 -> [w40]
    shift-right: [w31] -> _
    shift-left: w3 -> [w46]
    shift-right: [w30] -> _
    shift-left: w2 -> [w45]
    shift-right: [w38] -> _
    shift-left: w1 -> [w43]
    tunnel: "3D Curve" -> [w39]
    shift-right: [w37] -> _
    shift-left: _ -> [w36]
    tunnel: w11 -> [w34]
    tunnel: w10 -> [w33]
    stop <- w42 stop-if-true
    n12 = event shown="[0] \"Fit!\": Value Change" {
      selector: _ -> [_ _ _]
      dyn-events: _ -> [_ _ _]
      timeout: w41 -> [_ _ _]
      tunnel: w49 -> [w69 _ w83]
      tunnel: w48 -> [w68 _ w82]
      tunnel: w47 -> [w66 _ w87]
      tunnel: w46 -> [w57 _ w78]
      tunnel: w45 -> [w56 _ w77]
      tunnel: w44 -> [w63 _ w86]
      tunnel: w43 -> [w54 _ w76]
      tunnel: [_ "stop" _] -> w42
      tunnel: w40 -> [w64 _ w88]
      tunnel: w39 -> [w51 _ w84]
      tunnel: [w57 _ w78] -> w31
      tunnel: [w56 _ w77] -> w30
      tunnel: [w54 _ w76] -> w38
      tunnel: [w58 _ "Guess"] -> w37
      tunnel: w36 -> [w58 _ _]
      tunnel: [w59 _ _] -> w35
      tunnel: w34 -> [_ _ _]
      tunnel: w33 -> [_ _ _]
      tunnel: [w52 _ w90] -> w29
      tunnel: [w50 _ _] -> w27
      event "Fit!": Value Change {
        # "calculates best fit and updates\ngraph accordingly"
        # "Recalculate surface\nwith best fit paramters"
        n13 = event-data() -> ()  [unwired: 1 in, 1 out]
        n14 = Interleave 1D Arrays(w57, w56) -> (w65:dbl[])
        n15 = call-poly <vilib>:"Nonlinear Curve Fit.vi"("Y"=w54, "f(x,a)"=w64, "X"=w65, "initial parameters"=w58) -> ("best nonlinear fit"=w53:dbl[], "best fit parameters"=w50:dbl[], "error out"=w61:errorcluster)  [unwired: 6 in, 3 out]
        n16 = Unbundle By Name(w61) -> ("code"=w60:i32)
        n17 = call-by-ref "?"(reference=w64, "X"=w63, "Coefficients"=w50) -> ("f(X,a)"=w62:dbl[])  [unwired: 3 in, 4 out]
        n18 = case shown="0" w60 {
          selector: w60 -> [w73 _]
          tunnel: [w72 "Fit succeeded!"] -> w59
          frame Default {
            n19 = Format Into String(format string="Fit failed with error code: %d", w73) -> (resulting string=w72:string)  [unwired: 2 in, 1 out]
          }
          frame 0 {
          }
        }
        n20 = Reshape Array(w62, w66, w66) -> (w67:dbl[][])
        n21 = call <vilib>:"3D Surface.vi"("plot number (1)"=2, "z matrix"=w67, "y vector"=w68, "x vector"=w69, "3D graph"=w51) -> ()  [unwired: 5 in, 2 out]
        n22 = Subtract(x=w54, y=w53) -> (x-y=w55:dbl[])
        n23 = Build Array(w54, w53, w55) -> (w52:dbl[][])
      }
      event "stop": Value Change {
        n24 = event-data() -> ()  [unwired: 1 in, 1 out]
      }
      event "Guess": Value Change; Timeout {
        # "Any chage in input parameters clears the best fit\nand shows the best guess surface"
        n25 = event-data() -> ()  [unwired: 1 in, 1 out]
        n26 = call-by-ref "?"(reference=w88, "X"=w86, "Coefficients"="Guess") -> ("f(X,a)"=w89:dbl[])  [unwired: 3 in, 4 out]
        n27 = Reshape Array(w89, w87, w87) -> (w81:dbl[][])
        n28 = call <vilib>:"3D Surface.vi"("plot number (1)"=2, "z matrix"=w81, "y vector"=w82, "x vector"=w83, "3D graph"=w84) -> ("3D graph out"=w80:refnum<k7>)  [unwired: 5 in, 1 out]
        n29 = Interleave 1D Arrays(w78, w77) -> (w91:dbl[])
        n30 = call <vilib>:"3D Curve.vi"("plot number (1)"=1, "z vector"=w76, "y vector"=w77, "x vector"=w78, "3D graph"=w80) -> ()  [unwired: 5 in, 2 out]
        n31 = call-by-ref "?"(reference=w88, "X"=w91, "Coefficients"="Guess") -> ("f(X,a)"=w92:dbl[])  [unwired: 3 in, 4 out]
        n32 = Build Array(w76, w92) -> (w90:dbl[][])
      }
    }
    "note" <- w35
    "Z, Fit/Guess, Residual" <- w29
    "Best Fit" <- w27
    n33 = Build Array(w31, w30) -> (→"X,Y":dbl[][])
  }
